vi "getStatus.vi"(8 "error in (no error)":errorcluster, 9 "Monochromator in":refnum<class "Monochromator.lvclass">, 11 "ReadySate in":refnum<class "ReadySate.lvclass">) -> (0 "error out":errorcluster, 1 "Monochromator out":refnum<class "Monochromator.lvclass">, 3 "ReadySate out":refnum<class "ReadySate.lvclass">)   [LabVIEW 2016, in "ReadySate.lvclass"]
uses:
  ReadySate.lvclass
  Monochromator/Monochromator.lvclass
  Typedefs/DeviceStatus.ctl
  Monochromator/Monochromator.lvclass/Monochromator.ctl
  MonoCommunicator/MonoCommunicator.lvclass
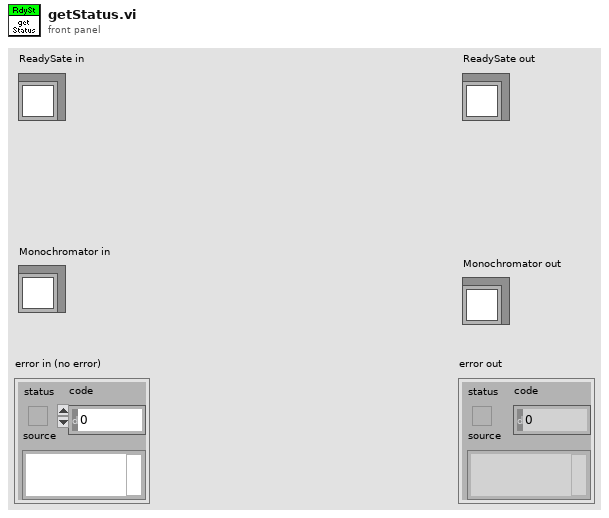
[diagram p1: front panel]
types:
  T1 = typedef "DeviceStatus.ctl" = enum16{"SettingUp", "Ready", "Offline", "Fault"}
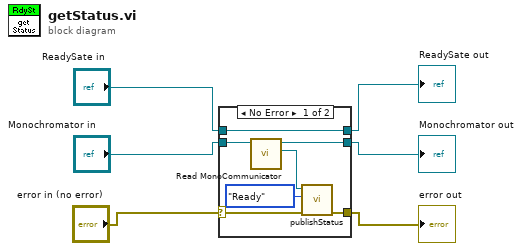
[diagram p0: block diagram]
diagram:
  n1 = case shown="No Error" "error in (no error)" {
    selector: "error in (no error)" -> [w8 w16]
    tunnel: [w9 w16] -> w5
    tunnel: [w13 w15] -> w4
    tunnel: "ReadySate in" -> [w13 w15]
    tunnel: [w12 w14] -> w1
    tunnel: "Monochromator in" -> [w11 w14]
    frame No Error {
      n2 = call "Read MonoCommunicator.vi"("Monochromator in"=w11) -> ("MonoCommunicator.lvclass"=w10:refnum<class "MonoCommunicator.lvclass">, "Monochromator out"=w12:refnum<class "Monochromator.lvclass">)  [unwired: 8 in, 1 out]
      n3 = call "publishStatus.vi"("error in (no error)"=w8, "DeviceStatus"=DeviceStatus."Ready", "MonoCommunicator in"=w10) -> ("error out"=w9:errorcluster)  [unwired: 7 in, 1 out]
    }
    frame Error {
    }
  }
  "error out" <- w5
  "ReadySate out" <- w4
  "Monochromator out" <- w1
